vi "Untitled 11 (SubVI).vi"(9 "Recorded T (K)":dbl, 10 "Min T(K)":dbl, 11 "Max T (K)":dbl) -> (1 "SHUTDOWN IS REQUIRED":bool, 2 "DILUATION IS REQUIRED":bool, 3 "COOLING IS ENOUGH":bool, 4 "String":string)   [LabVIEW 2019]
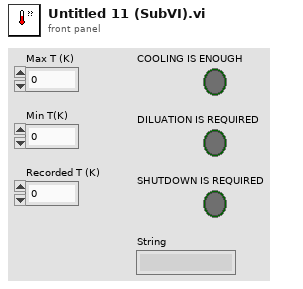
[diagram p1: front panel]
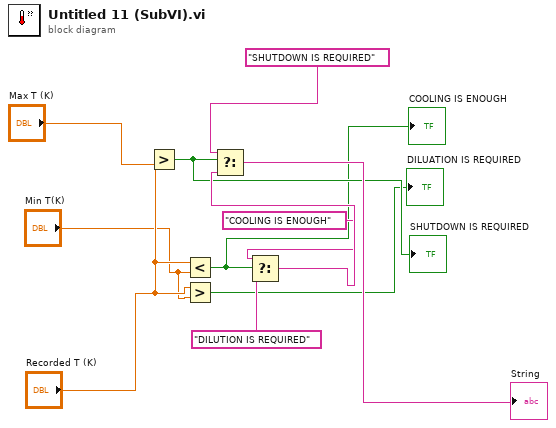
[diagram p0: block diagram]
diagram:
  n1 = Greater?(x="Recorded T (K)", y="Max T (K)") -> (0:w6:bool)
  "SHUTDOWN IS REQUIRED" <- w6
  n2 = Less?(x="Recorded T (K)", y="Min T(K)") -> (x < y?=w1:bool)
  "COOLING IS ENOUGH" <- w1
  n3 = Greater?(x="Recorded T (K)", y="Min T(K)") -> (0:→"DILUATION IS REQUIRED":bool)
  n4 = Select(t="COOLING IS ENOUGH", s=w1, f="DILUTION IS REQUIRED") -> (s? t:f=w10:string)
  n5 = Select(t="SHUTDOWN IS REQUIRED", s=w6, f=w10) -> (s? t:f=→"String":string)
